vi "get unmapped tag list.vi"(11 "engine configuration in":refnum<class "engine configuration.lvclass">) -> (2 "tag list":refnum<class "tag descriptor.lvclass">[](array[class]), 3 "engine configuration out":refnum<class "engine configuration.lvclass">)   [LabVIEW 2013, in "engine configuration.lvclass"]
doc: "Reads all tags which have no reading channel and no writing channel."
uses:
  engine configuration.lvclass
  <vilib>/NI/Tag Bus/tag/tag descriptor.lvclass
  engine configuration.lvclass/engine configuration.ctl
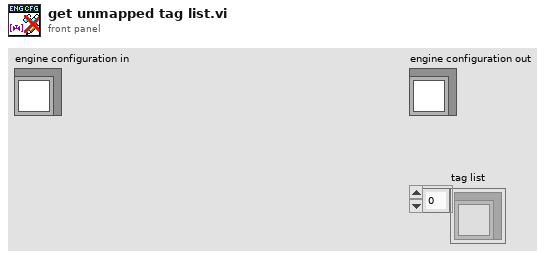
[diagram p1: front panel]
types:
  T1 = typedef "engine configuration.lvclass/module channel pairings.ctl" = cluster{"modules":string[], "channels":string[]}
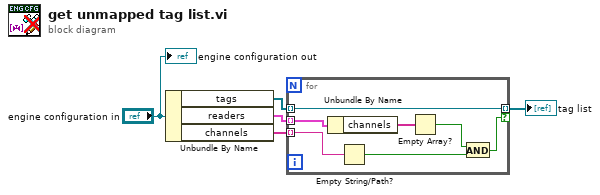
[diagram p0: block diagram]
diagram:
  n1 = Unbundle By Name("engine configuration in") -> ("tags"=w4:refnum<class "tag descriptor.lvclass">[], "readers"=w2:T1[], "channels"=w1:string[])
  n2 = for {
    tunnel: w4 -> [w12] mode=indexing
    tunnel: [w12] -> w3 mode=indexing if=w6
    tunnel: w2 -> [w11] mode=indexing
    tunnel: w1 -> [w8] mode=indexing
    n3 = Unbundle By Name(w11) -> ("channels"=w10:string[])
    n4 = Empty String/Path?(string/path=w8) -> (empty?=w7:bool)
    n5 = Empty Array?(array=w10) -> (empty?=w9:bool)
    n6 = And(x=w9, y=w7) -> (x .and. y?=w6:bool)
  }
  "tag list" <- w3
  "engine configuration out" <- "engine configuration in"
